vi "Create Default Line.vi"() -> ()   [LabVIEW 2017, in "J1939 configuration.lvclass"]
uses:
  J1939 configuration.lvclass
  Line.ctl
  <vilib>/NI/Tag Bus Module Framework/channel/TBM channel.lvclass
panel:
  in  "Line":T1={"channel"=refnum, "XNET Signal"="CANEventSignal1\nNIXNET_example.CAN_Cluster"}
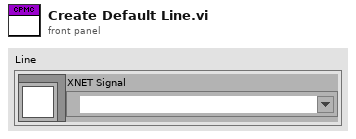
[diagram p1: front panel]
types:
  T1 = typedef "J1939 configuration.lvclass/Line.ctl" = cluster{"channel":refnum<class "TBM channel.lvclass">, "XNET Signal":refnum<k21>}
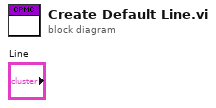
[diagram p0: block diagram]
diagram:
